vi "ByValue1_Init.vi"(8 "error in (no error)":errorcluster, 10 "ProgressTrigger":refnum<vi>, 11 "object in":refnum<class "ByValue1.lvclass">) -> (0 "error out":errorcluster, 3 "object out":refnum<class "ByValue1.lvclass">)   [LabVIEW 2020, in "ByValue1.lvclass"]
uses:
  ByValue1.lvclass
  ByValue1.lvclass/ByValue1.ctl
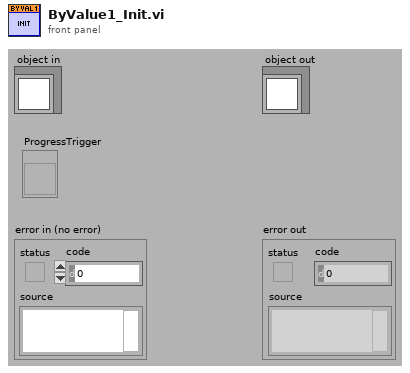
[diagram p1: front panel]
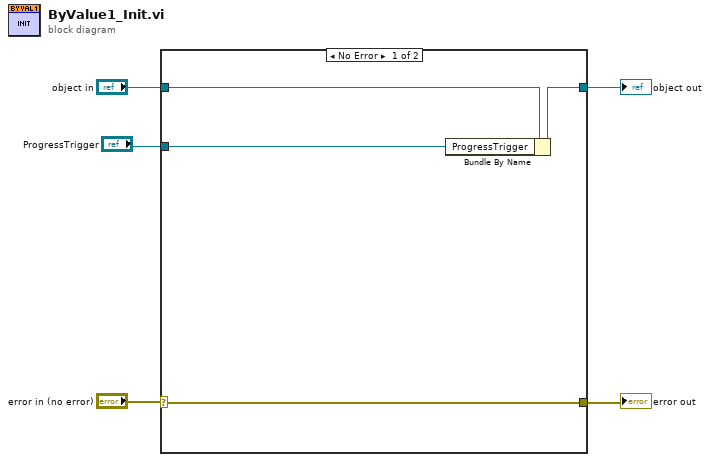
[diagram p0: block diagram]
diagram:
  n1 = case shown="No Error" "error in (no error)" {
    selector: "error in (no error)" -> [w7 w10]
    tunnel: "object in" -> [w9 w11]
    tunnel: [w8 w11] -> w4
    tunnel: [w7 w10] -> w2
    tunnel: "ProgressTrigger" -> [w6 _]
    frame No Error {
      n2 = Bundle By Name(cluster=w9, "ProgressTrigger"=w6) -> (w8:refnum<class "ByValue1.lvclass">)
    }
    frame Error {
    }
  }
  "object out" <- w4
  "error out" <- w2
